vi "Merge Managers.vi"(10 "ConfigManager B":refnum<class "ConfigManager.lvclass">, 11 "ConfigManager A":refnum<class "ConfigManager.lvclass">) -> (3 "ConfigManagerCollection":refnum<class "ConfigManagerCollection.lvclass">)   [LabVIEW 2013, in "SMOConfig.lvlib" / "ConfigManager.lvclass"]
uses:
  ConfigManager.lvclass
  Collection/ConfigManagerCollection.lvclass
  Cache/ConfigManager.Cache.lvclass
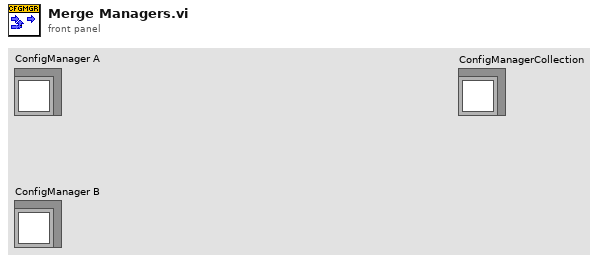
[diagram p1: front panel]
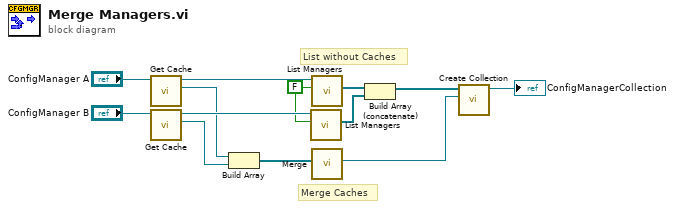
[diagram p0: block diagram]
diagram:
  w1 = FALSE ("Include Cache? (F)")
  # "Merge Caches"
  # "List without Caches"
  n1 = call-dynamic "Get Cache.vi"("ConfigManager in"="ConfigManager A") -> ("Cache"=w5:refnum<class "ConfigManager.Cache.lvclass">, "ConfigManager out"=w8:refnum<class "ConfigManager.lvclass">)  [unwired: 8 in, 1 out]
  n2 = call-dynamic "Get Cache.vi"("ConfigManager in"="ConfigManager B") -> ("Cache"=w4:refnum<class "ConfigManager.Cache.lvclass">, "ConfigManager out"=w6:refnum<class "ConfigManager.lvclass">)  [unwired: 8 in, 1 out]
  n3 = Build Array(w5, w4) -> (w3:refnum<class "ConfigManager.Cache.lvclass">[])
  n4 = call-dynamic "List Managers.vi"("Include Cache? (F)"=w1, "SMOConfigManager in"=w6) -> ("List"=w13:refnum<class "ConfigManager.lvclass">[])  [unwired: 8 in, 1 out]
  n5 = call-dynamic "List Managers.vi"("Include Cache? (F)"=w1, "SMOConfigManager in"=w8) -> ("List"=w12:refnum<class "ConfigManager.lvclass">[])  [unwired: 8 in, 1 out]
  n6 = call "Merge.vi"("Cache Managers"=w3) -> ("Merged Cache"=w2:refnum<class "ConfigManager.Cache.lvclass">)  [unwired: 10 in]
  n7 = Build Array (concatenate)(w12, w13) -> (w11:refnum<class "ConfigManager.lvclass">[])
  n8 = call "Create Collection.vi"("Cache"=w2, "List"=w11) -> ("SMOConfigManagerCollection out"=→"ConfigManagerCollection":refnum<class "ConfigManagerCollection.lvclass">)  [unwired: 9 in]
